vi "Write Physical Address.vi"(10 "Physical Address":u32, 11 "Toggle 6 in":refnum<class "Toggle 6.lvclass">) -> (3 "Toggle 6 out":refnum<class "Toggle 6.lvclass">)   [LabVIEW 2020, in "Toggle 6.lvclass"]
uses:
  Toggle 6.lvclass
  Toggle 6.lvclass/Toggle 6.ctl
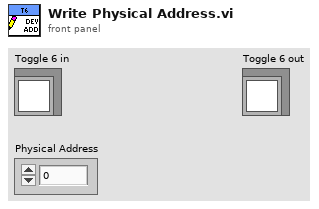
[diagram p1: front panel]
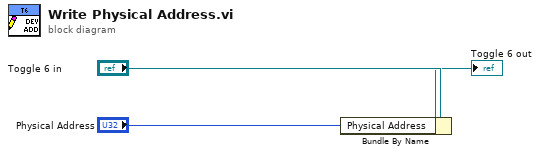
[diagram p0: block diagram]
diagram:
  n1 = Bundle By Name(cluster="Toggle 6 in", "Physical Address"="Physical Address") -> (→"Toggle 6 out":refnum<class "Toggle 6.lvclass">)
